vi "Get all VI references.vi"(8 "error in (no error)":errorcluster, 11 "Project Item":refnum<vi>) -> (0 "error out":errorcluster, 3 "VI Refs":refnum<vi>[](array[refnum]))   [LabVIEW 2015]
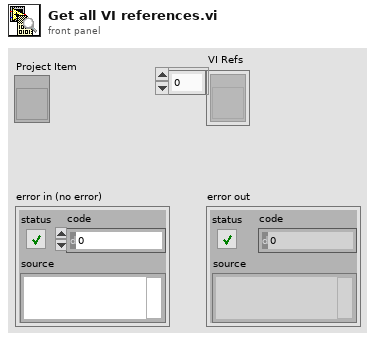
[diagram p1: front panel]
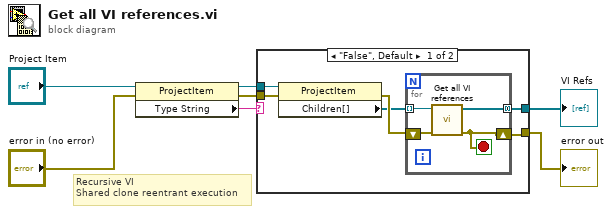
[diagram p0: block diagram]
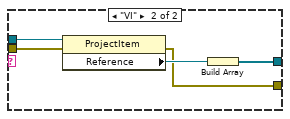
[diagram p2: hidden frame]
diagram:
  # "Recursive VI\nShared clone reentrant execution"
  n1 = property class="ProjectItem"(reference="Project Item", error in="error in (no error)") -> (reference out=w5:refnum<vi>, error out=w4:errorcluster, "Type String"=w6:string)
  n2 = case shown="\"False\", Default" w6 {
    tunnel: w5 -> [w13 w22]
    tunnel: w4 -> [w11 w21]
    tunnel: [w8 w19] -> w1
    tunnel: [w9 w18] -> w2
    frame "False", Default {
      n3 = property class="ProjectItem"(reference=w13, error in=w11) -> (error out=w12:errorcluster, "Children[]"=w10:refnum<vi>[])  [unwired: 1 out]
      n4 = for {
        tunnel: w10 -> [w17] mode=indexing
        shift-right: [w15] -> w9
        shift-left: w12 -> [w16]
        tunnel: [w14] -> w8 mode=concatenating
        stop <- w15 stop-if-true
        n5 = call "Get all VI references.vi"("error in (no error)"=w16, "Project Item"=w17) -> ("error out"=w15:errorcluster, "VI Refs"=w14:refnum<vi>[])  [unwired: 8 in]
      }
    }
    frame "VI" {
      n6 = property class="ProjectItem"(reference=w22, error in=w21) -> (error out=w18:errorcluster, "Reference"=w20:refnum<vi>)  [unwired: 1 out]
      n7 = Build Array(w20) -> (w19:refnum<vi>[])
    }
  }
  "error out" <- w2
  "VI Refs" <- w1
